vi "SSL Ref.vi"(6 "Action":T1, 8 "Error In":errorcluster, 11 "SSL Stream":refnum<k24>) -> (0 "Error Out":errorcluster, 3 "SSL Stream":refnum<k24>)   [LabVIEW 2014, in "SSL Lib.lvlib"]
doc: "VI Function: This is a Functional Global that stores the SSL stream reference.\n\nVI Version: 1.0\n\nVI Author: Runjhun Agarwal"
uses:
  <userlib>/SSL Library/SSL Lib.lvlib
  <userlib>/SSL Library/Controls/Ref.ctl
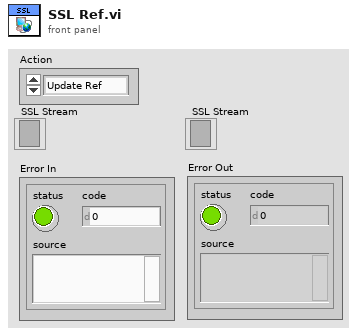
[diagram p1: front panel]
types:
  T1 = typedef "Ref.ctl" = enum16{"Update Ref", "Read Ref", "Close Ref"}
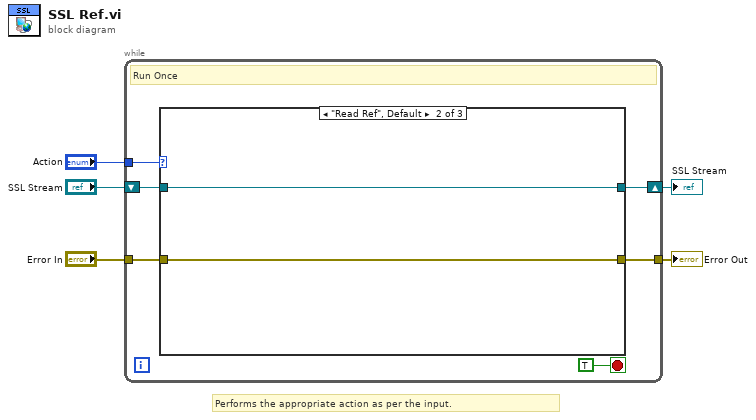
[diagram p0: block diagram]
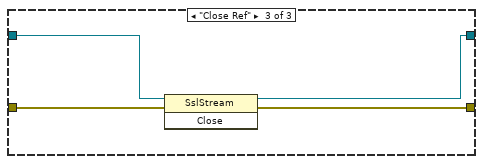
[diagram p3: hidden frame]
diagram:
  # "Performs the appropriate action as per the input."
  n1 = while {
    tunnel: "Action" -> [w10]
    shift-right: [w8] -> w2
    shift-left: "SSL Stream" -> [w9]
    tunnel: "Error In" -> [w7]
    tunnel: [w6] -> w3
    stop <- TRUE stop-if-true
    # "Run Once"
    n2 = case shown="\"Read Ref\", Default" w10 {
      tunnel: w9 -> [w12 w15 w19]
      tunnel: [w12 w15 w16] -> w8
      tunnel: w7 -> [w13 w14 w18]
      tunnel: [w13 w14 w17] -> w6
      frame "Update Ref" {
      }
      frame "Read Ref", Default {
      }
      frame "Close Ref" {
        n3 = invoke class="SslStream" method="Close"(reference=w19, error in=w18) -> (reference out=w16:refnum<k24>, error out=w17:errorcluster)  [unwired: 1 in, 1 out]
      }
    }
  }
  "Error Out" <- w3
  "SSL Stream" <- w2
